vi "DMD_flippityfloppity.vi"() -> ()   [LabVIEW 2017]
panel:
  in  "stop":bool
  in  "milliseconds to wait":u32=100
  in  "String 2":string="C:\\Users\\1TEM\\Documents\\MATLAB\\MASKS\\UP.bmp"
  in  "String":string="C:\\Users\\1TEM\\Documents\\MATLAB\\MASKS\\DOWN.bmp"
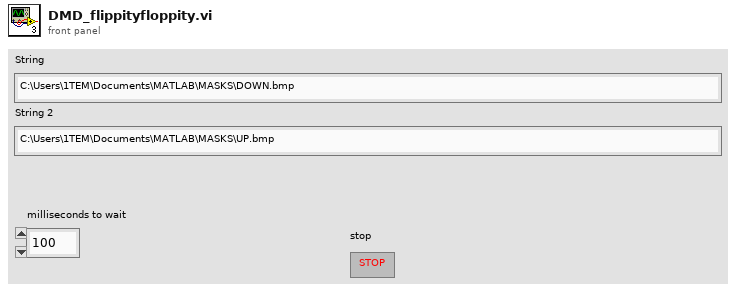
[diagram p1: front panel]
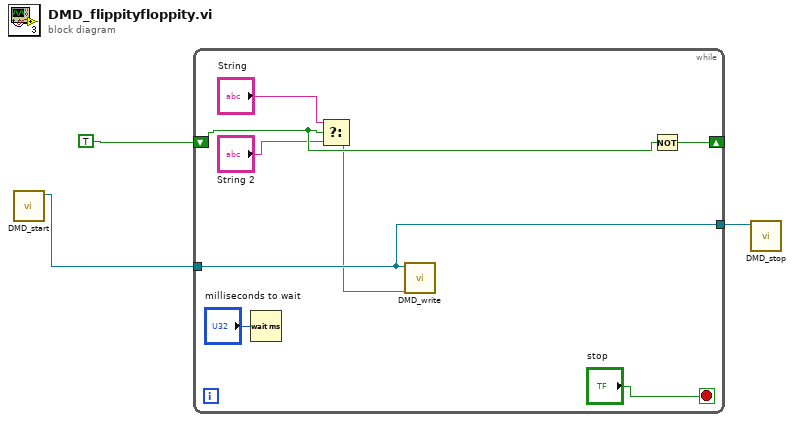
[diagram p0: block diagram]
diagram:
  n1 = call "DMD_start.vi"() -> ("reference out"=w2:refnum<k24>)  [unwired: 10 in, 1 out]
  n2 = while {
    shift-right: [w10] -> _
    shift-left: TRUE -> [w11]
    tunnel: w2 -> [w6]
    tunnel: [w6] -> w1
    stop <- "stop" stop-if-true
    n3 = Wait (ms)(milliseconds to wait="milliseconds to wait") -> ()  [unwired: 1 out]
    n4 = Select(t="String", s=w11, f="String 2") -> (s? t:f=w5:string)
    n5 = call "DMD_write.vi"("String"=w5, "reference out"=w6) -> ()  [unwired: 9 in, 1 out]
    n6 = Not(x=w11) -> (.not. x?=w10:bool)
  }
  n7 = call "DMD_stop.vi"("reference out"=w1) -> ()  [unwired: 10 in, 1 out]
